vi "mediaRobos_v2.vi"(10 "Field Size 2":T2, 11 "Array Robot Pose + CamID":T1(array[cluster])) -> (3 "Array":cluster{"x":dbl, "y":dbl, "robot_id":i32}[](array[cluster]))   [LabVIEW 2018]
panel:
  in  "file path (use dialog) 2":path=path "C:/Users/RoboIme/git/sslview/Util/Farias2.csv"
  in  "cluster":cluster{"x":dbl, "y":dbl, "robot_id":i32}
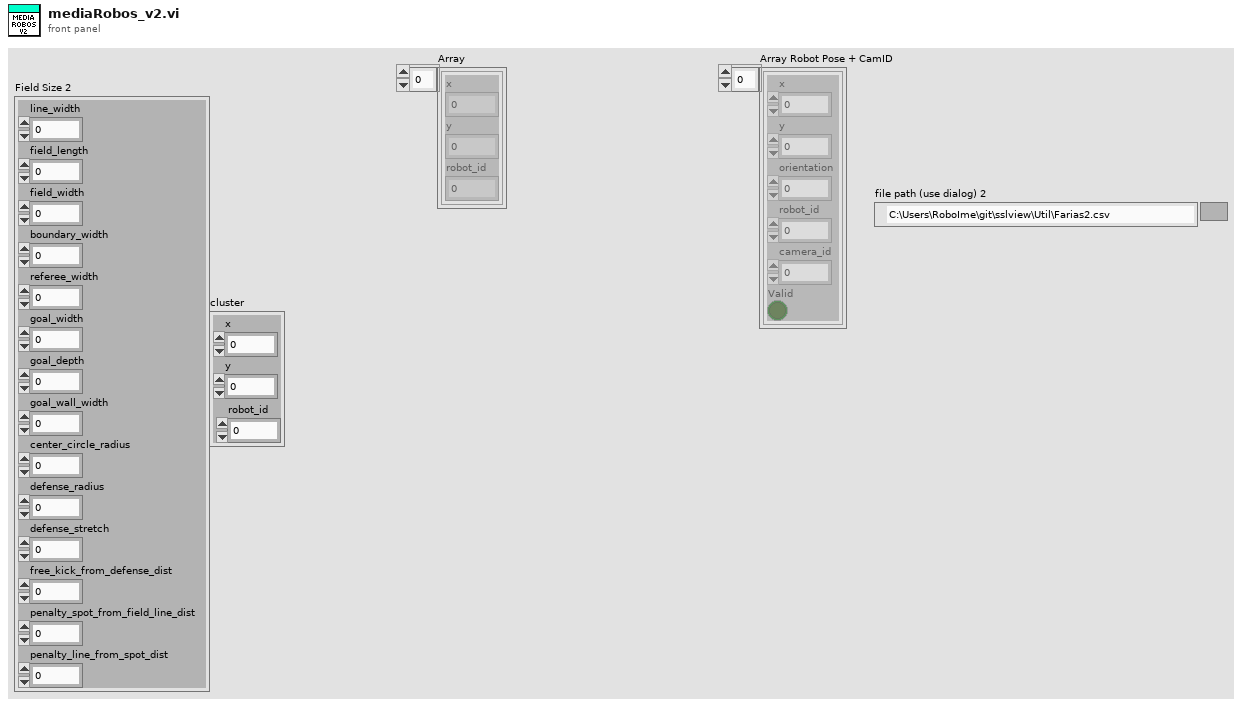
[diagram p1: front panel]
types:
  T1 = cluster{"x":sgl, "y":sgl, "orientation":sgl, "robot_id":u32, "camera_id":u32, "Valid":bool}[]
  T2 = cluster{"line_width":u32, "field_length":u32, "field_width":u32, "boundary_width":u32, "referee_width":u32, "goal_width":u32, "goal_depth":u32, "goal_wall_width":u32, "center_circle_radius":u32, "defense_radius":u32, "defense_stretch":u32, "free_kick_from_defense_dist":u32, "penalty_spot_from_field_line_dist":u32, "penalty_line_from_spot_dist":u32}
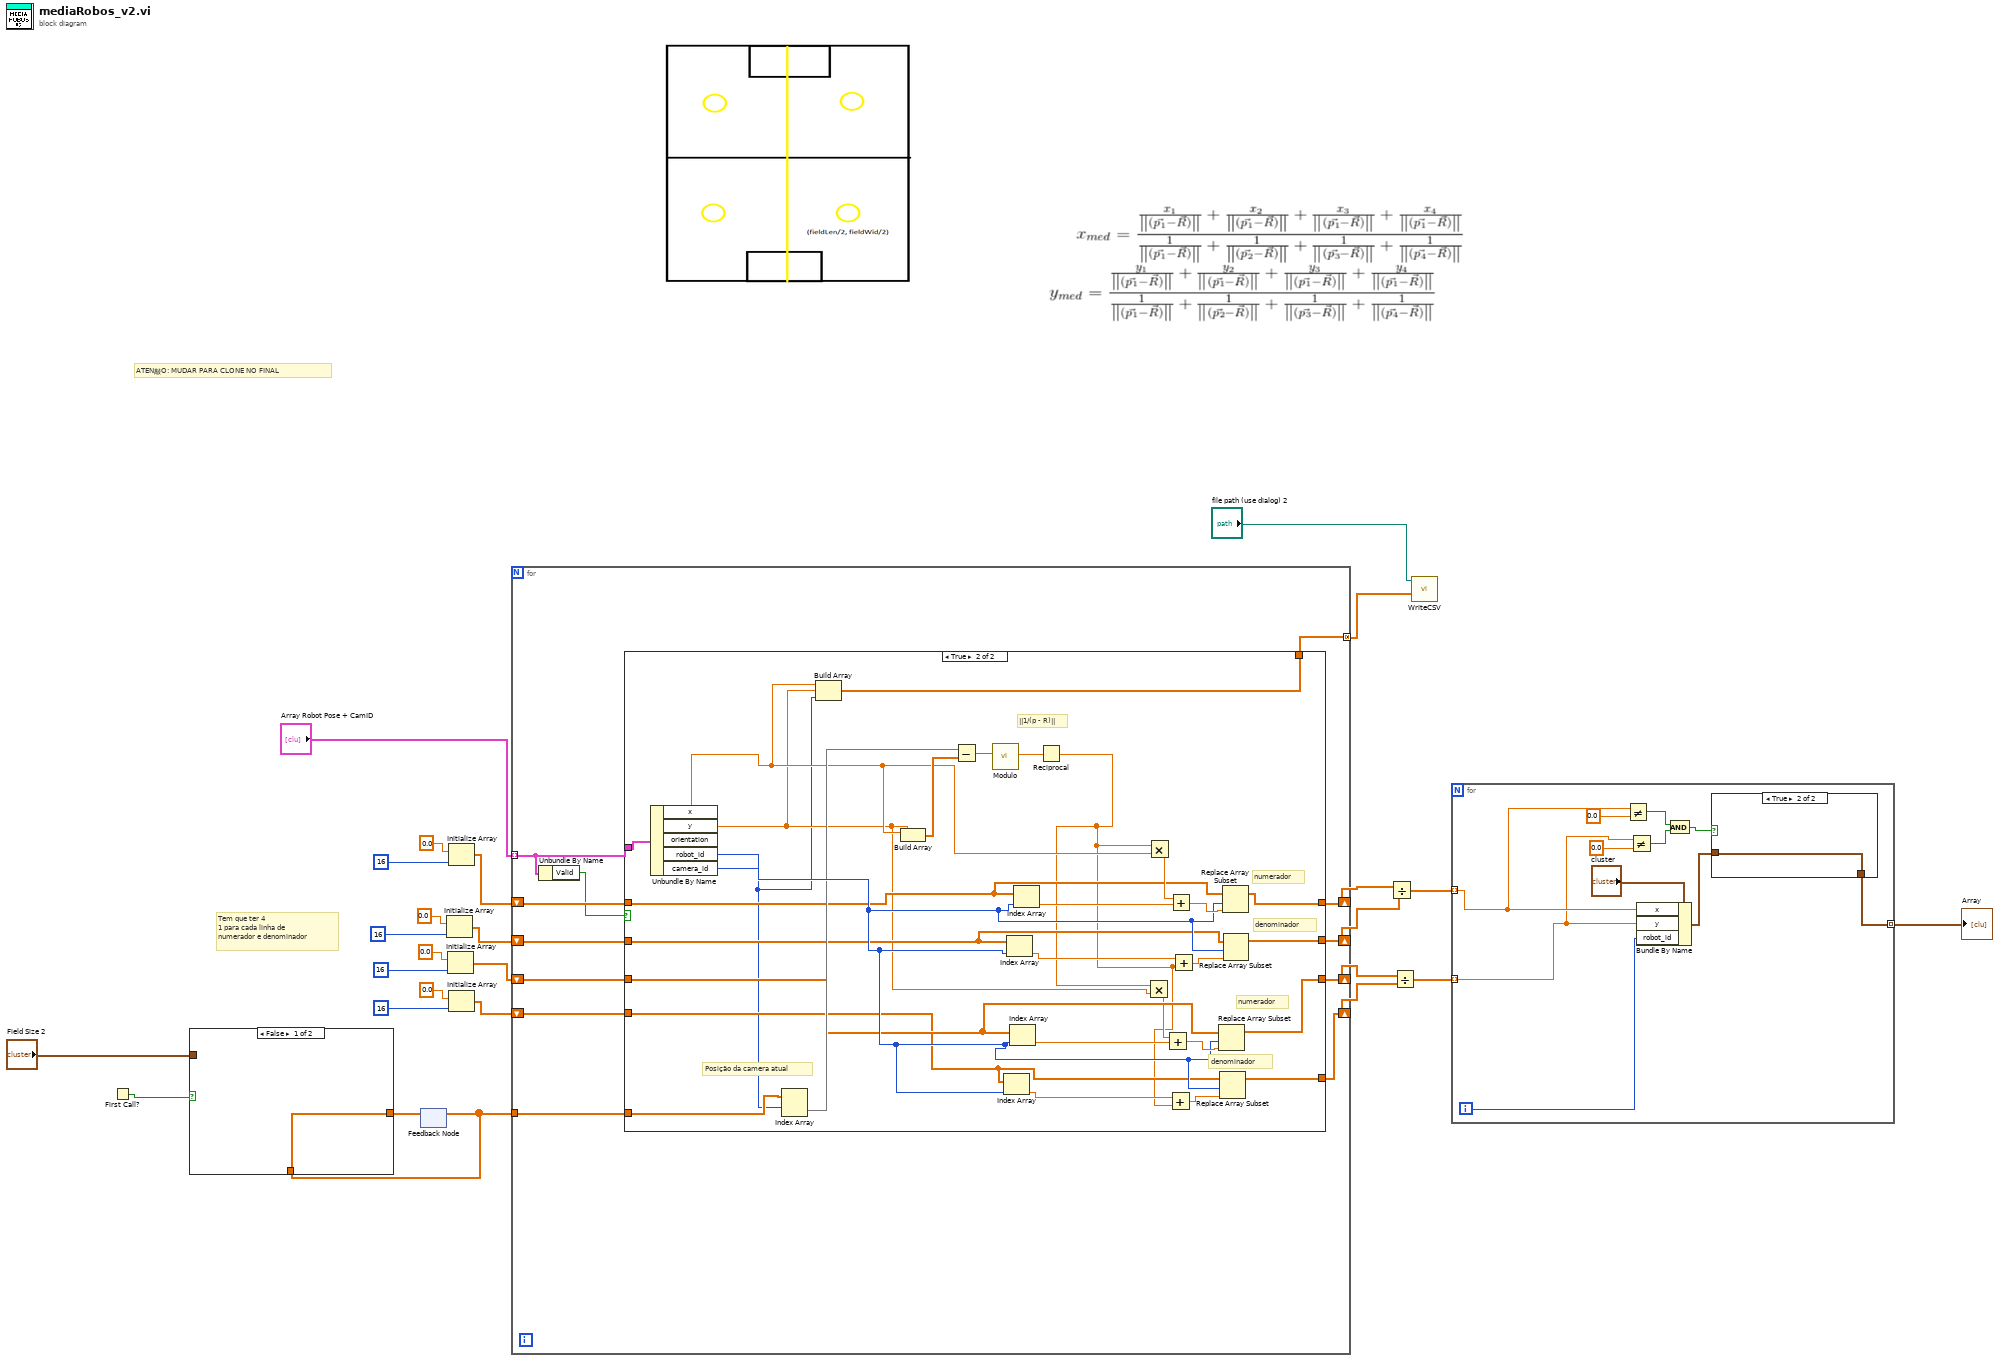
[diagram p0: block diagram]
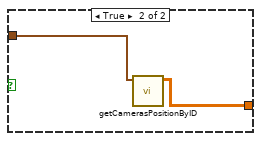
[diagram p2: hidden frame]
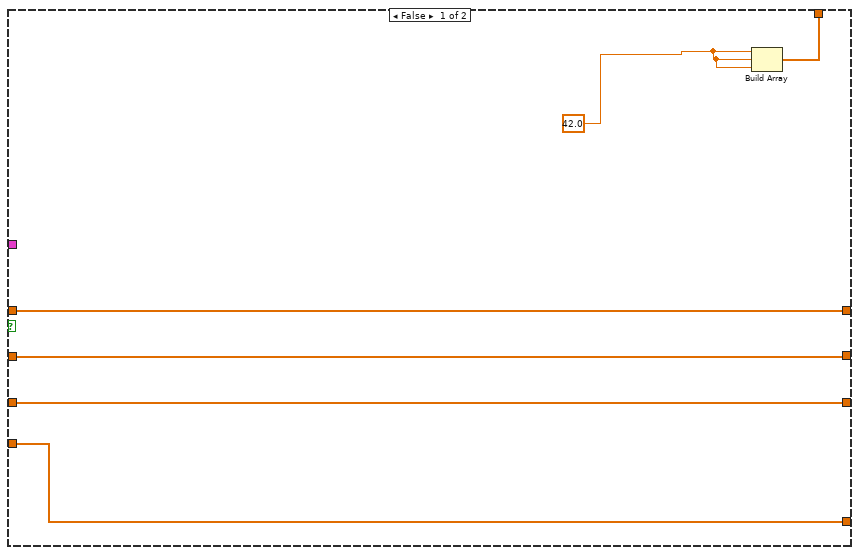
[diagram p4: hidden frame]
diagram:
  # "Tem que ter 4\n1 para cada linha de\nnumerador e denominador"
  # "ATEN敲O: MUDAR PARA CLONE NO FINAL"
  n1 = First Call?() -> (First Call?: T/F=w3:bool)
  n2 = feedback #1() -> (w1:dbl[][])  [unwired: 1 in]
  n3 = case shown="False" w3 {
    tunnel: "Field Size 2" -> [_ w29]
    tunnel: [w27 w28] -> w2
    tunnel: w1 -> [w27 _]
    frame False {
    }
    frame True {
      n4 = call "getCamerasPositionByID.vi"("Field Size 2"=w29) -> ("Cameras Positions"=w28:dbl[][])  [unwired: 10 in]
    }
  }
  n5 = feedback-in #1(w2) -> ()
  n6 = Initialize Array(0.0 ("element"), 16 ("dimension size")) -> (w17:dbl[])
  n7 = Initialize Array(0.0 ("element"), 16 ("dimension size")) -> (w16:dbl[])
  n8 = Initialize Array(0.0 ("element"), 16 ("dimension size")) -> (w18:dbl[])
  n9 = Initialize Array(0.0 ("element"), 16 ("dimension size")) -> (w15:dbl[])
  n10 = for {
    tunnel: "Array Robot Pose + CamID" -> [w31] mode=indexing
    tunnel: w1 -> [w41]
    shift-right: [w40] -> w14
    shift-left: w18 -> [w34]
    shift-right: [w39] -> w13
    shift-left: w17 -> [w33]
    shift-right: [w38] -> w12
    shift-left: w16 -> [w36]
    shift-right: [w37] -> w11
    shift-left: w15 -> [w35]
    tunnel: [w32] -> w6 mode=concatenating
    n11 = Unbundle By Name(w31) -> ("Valid"=w30:bool)
    n12 = case shown="True" w30 {
      tunnel: w31 -> [_ w77]
      tunnel: w41 -> [_ w76]
      tunnel: [w47 w61] -> w40
      tunnel: [w46 w60] -> w39
      tunnel: [w45 w59] -> w38
      tunnel: [w44 w58] -> w37
      tunnel: w36 -> [w45 w57]
      tunnel: w35 -> [w44 w56]
      tunnel: w34 -> [w47 w55]
      tunnel: w33 -> [w46 w54]
      tunnel: [w43 w49] -> w32
      frame False {
        w42 = 42.0 ("element")
        n13 = Build Array(w42, w42, w42) -> (w43:dbl[])
      }
      frame True {
        # "denominador"
        # "numerador"
        # "denominador"
        # "numerador"
        # "||1/(p - R)||"
        # "Posição da camera atual"
        n14 = Unbundle By Name(w77) -> ("x"=w52:sgl, "y"=w51:sgl, "robot_id"=w67:u32, "camera_id"=w50:u32)  [unwired: 1 out]
        n15 = Index Array(array=w76, index (row)=w50) -> (element=w66:dbl[])  [unwired: 1 in]
        n16 = Build Array(w52, w51, w50) -> (w49:sgl[])
        n17 = Build Array(w52, w51) -> (w75:sgl[])
        n18 = Subtract(x=w66, y=w75) -> (x-y=w74:dbl[])
        n19 = call "Modulo.vi"("2D vector"=w74) -> ("Modulo"=w73:dbl)  [unwired: 10 in]
        n20 = Index Array(array=w56, index=w67) -> (element=w62:dbl)
        n21 = Index Array(array=w54, index=w67) -> (element=w64:dbl)
        n22 = Index Array(array=w57, index=w67) -> (element=w63:dbl)
        n23 = Index Array(array=w55, index=w67) -> (element=w65:dbl)
        n24 = Reciprocal(x=w73) -> (1/x=w48:dbl)
        n25 = Multiply(x=w48, y=w51) -> (x*y=w53:dbl)
        n26 = Multiply(x=w48, y=w52) -> (x*y=w72:dbl)
        n27 = Add(x=w53, y=w63) -> (x+y=w69:dbl)
        n28 = Add(x=w62, y=w48) -> (x+y=w68:dbl)
        n29 = Add(x=w72, y=w65) -> (x+y=w71:dbl)
        n30 = Add(x=w64, y=w48) -> (x+y=w70:dbl)
        n31 = Replace Array Subset(array=w57, new element=w69, index=w67) -> (w59:dbl[])
        n32 = Replace Array Subset(array=w56, new element=w68, index=w67) -> (w58:dbl[])
        n33 = Replace Array Subset(array=w55, new element=w71, index=w67) -> (w61:dbl[])
        n34 = Replace Array Subset(array=w54, new element=w70, index=w67) -> (w60:dbl[])
      }
    }
  }
  n35 = Divide(x=w14, y=w13) -> (x/y=w10:dbl[])
  n36 = Divide(x=w12, y=w11) -> (x/y=w9:dbl[])
  n37 = call "WriteCSV.vi"("array"=w6, "file path (use dialog)"="file path (use dialog) 2") -> ()  [unwired: 10 in]
  n38 = for {
    tunnel: w10 -> [w87] mode=indexing
    tunnel: w9 -> [w84] mode=indexing
    tunnel: [w80] -> w8 mode=indexing
    i -> [w88]
    n39 = Not Equal?(x=w87, y=0.0) -> (x != y?=w83:bool)
    n40 = Not Equal?(x=w84, y=0.0) -> (x != y?=w82:bool)
    n41 = Bundle By Name(cluster="cluster", "x"=w87, "y"=w84, "robot_id"=w88) -> (w79:cluster{"x":dbl, "y":dbl, "robot_id":i32})
    n42 = And(x=w83, y=w82) -> (x .and. y?=w81:bool)
    n43 = case shown="True" w81 {
      tunnel: [w89 w90] -> w80
      tunnel: w79 -> [w89 w90]
      frame False {
      }
      frame True {
      }
    }
  }
  "Array" <- w8
